vi "Read freq.vi"(8 "error in":errorcluster, 11 "MultiUsrp in":refnum<class "MultiUsrp.lvclass">) -> (0 "error out":errorcluster, 2 "freq":dbl, 3 "MultiUsrp out":refnum<class "MultiUsrp.lvclass">)   [LabVIEW 2023, in "uhd.lvlib" / "MultiUsrp.lvclass"]
uses:
  <userlib>/uhd/MultiUsrp/MultiUsrp.lvclass
  <userlib>/uhd/MultiUsrp/MultiUsrp.lvclass/MultiUsrp.ctl
  <userlib>/uhd/uhd.lvlib
  <userlib>/uhd/usrp session.ctl
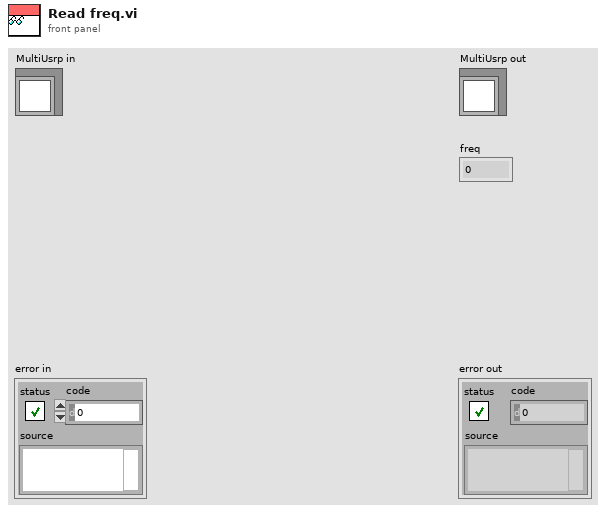
[diagram p1: front panel]
types:
  T1 = typedef "usrp session.ctl" = cluster{"h":u64, "Enum":enum16{"usrp handle"}}
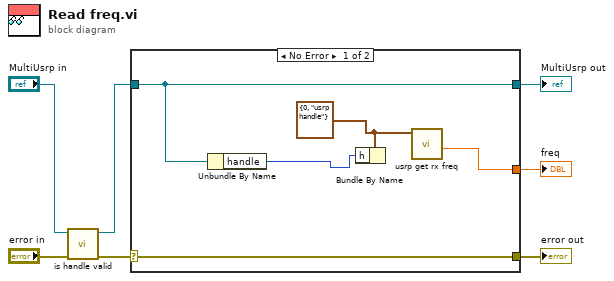
[diagram p0: block diagram]
diagram:
  n1 = call <userlib>:"is handle valid.vi"("error in (no error)"="error in", "MultiUsrp in"="MultiUsrp in") -> ("error out"=w1:errorcluster, "MultiUsrp out"=w2:refnum<class "MultiUsrp.lvclass">)  [unwired: 8 in]
  n2 = case shown="No Error" w1 {
    selector: w1 -> [w12 w13]
    tunnel: [w12 w13] -> w7
    tunnel: [w11 w14] -> w6
    tunnel: w2 -> [w11 w14]
    tunnel: [w8 _] -> w5
    frame No Error {
      w10 = T1 {"h"=0, "Enum"=enum."usrp handle"} ("h")
      n3 = Unbundle By Name(w11) -> ("handle"=w9:u64)
      n4 = Bundle By Name(cluster=w10, "h"=w9) -> ()  [unwired: 1 out]
      n5 = call <userlib>:"usrp get rx freq.vi"("h"=w10) -> ("freq_out out"=w8:dbl)  [unwired: 7 in, 3 out]
    }
    frame Error {
    }
  }
  "error out" <- w7
  "MultiUsrp out" <- w6
  "freq" <- w5
